vi "IOLINK LED STATE.vi"(7 "IP":string="192.168.23.100", 8 "error in (no error)":errorcluster) -> (0 "error out":errorcluster, 2 "MASTER STATUS":T2, 3 "JSON DATA - Payload":string)   [LabVIEW 2024]
uses:
  <vilib>/JDP Science/JSONtext/Find Item.vi
  <vilib>/JDP Science/JSONtext/String Subset.vi
  <vilib>/JDP Science/JSONtext/Offset/Find Object Item Locations by Names.vi
  <vilib>/JDP Science/JSONtext/support/Quote and Escape JSON string.vi
  <vilib>/JDP Science/JSONtext/Next JSON Value.vi
  <vilib>/JDP Science/JSONtext/Parsing/Advance past whitespace.vi
  <vilib>/JDP Science/JSONtext/support/Commas Needed.vi
  <vilib>/JDP Science/JSONtext/Parsing/Advance past whitespace and comma.vi
  <vilib>/JDP Science/JSONtext/Parsing/Advance past next JSON Value (inlined COPY).vi
  <vilib>/JDP Science/JSONtext/Parsing/Advance past Item Name.vi
  <vilib>/JDP Science/JSONtext/support/quote and escape json string 2.vi
  <vilib>/JDP Science/JSONtext/Parsing/Advance past Line Ending.vi
  <vilib>/JDP Science/JSONtext/Parsing/Advance past String.vi
  <vilib>/JDP Science/JSONtext/Parsing/Advance past Number.vi
  <vilib>/JDP Science/JSONtext/Parsing/Parse Full Path or Item Name.vi
  <vilib>/JDP Science/JSONtext/Parsing/Advance past Array.vi
  <vilib>/JDP Science/JSONtext/Parsing/Advance past Object.vi
  <vilib>/JDP Science/JSONtext/support/Error Cluster From Code.vi
  <vilib>/JDP Science/JSONtext/Offset/Find Item Locations by Path.vi
  <vilib>/JDP Science/JSONtext/Parsing/Parsing Error.vi
  <vilib>/JDP Science/JSONtext/JSONtext.lvlib
  <vilib>/NI/Advanced HTTP Client/Session.lvclass
panel:
  out "ON-offD 4":bool
  out "ON-offD 3":bool
  out "ON-offD 2":bool
  out "ON-offD":bool
  out "Statusd":bool
  out "Powerd":bool
  in  "MASTER STATUS 2":T1
  # "Master led status"
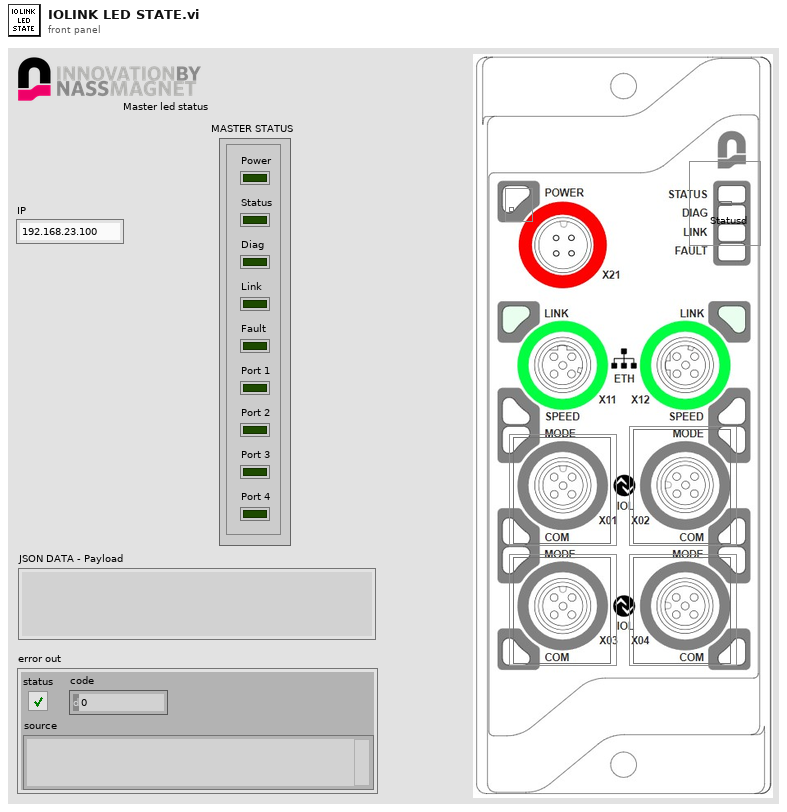
[diagram p1: front panel]
types:
  T1 = cluster{"Power":bool, "Status":bool, "Diag":bool, "Link":bool, "Fault":bool, "Port 1":bool, "Port 2":bool, "Port 3":bool, "Port 4":bool}
  T2 = cluster{"Power":bool, "Status":bool, "Diag":bool, "Link":bool, "Fault":bool, "Port 1":bool, "Port 3":bool, "Port 2":bool, "Port 4":bool}
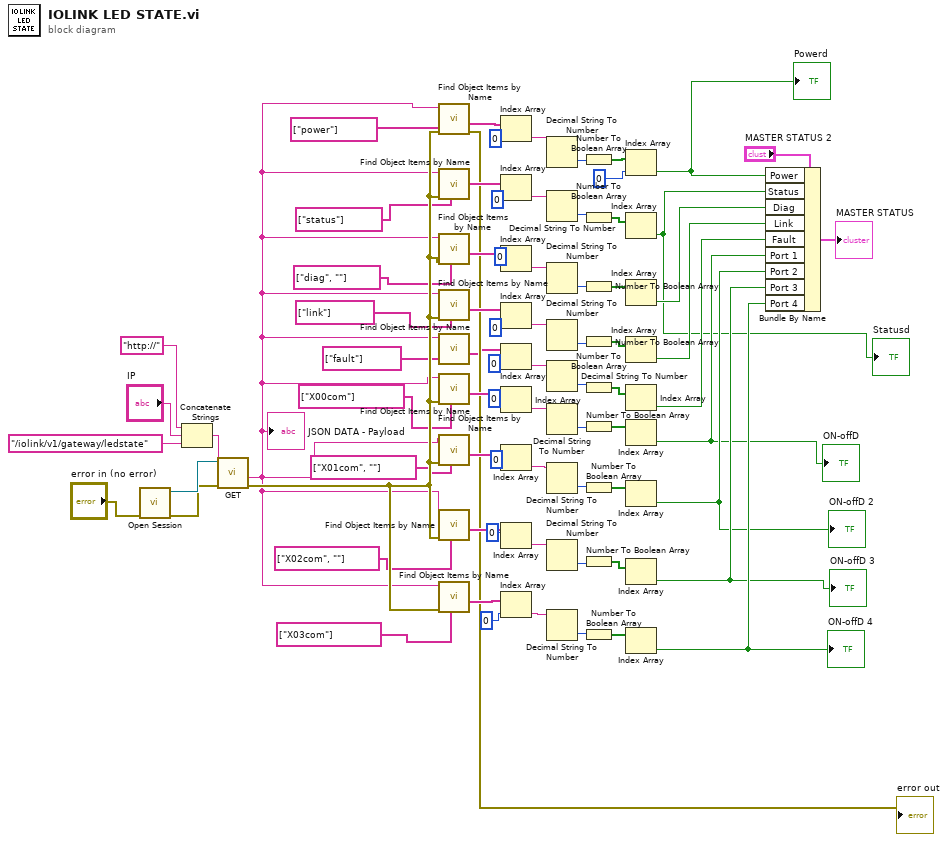
[diagram p0: block diagram]
diagram:
  n1 = call <vilib>:"Open Session.vi"("error in"="error in (no error)") -> ("error out"=w70:errorcluster, "session"=w72:refnum<class "Session.lvclass">)  [unwired: 9 in]
  n2 = Concatenate Strings("http://" ("url"), "IP", "/iolink/v1/gateway/ledstate" ("string")) -> (w71:string)
  n3 = call <vilib>:"GET.vi"("error in"=w70, "url"=w71, "session in"=w72) -> ("error out"=w66:errorcluster, "body"=w29:string)  [unwired: 4 in, 3 out]
  "JSON DATA - Payload" <- w29
  n4 = call <vilib>:"Find Object Items by Name.vi"("Item Names"=string[] ["power"], "error in (no error)"=w66, "JSON"=w29) -> ("error out"=→"error out":errorcluster, "<JSON>"=w69:string[])  [unwired: 6 in, 1 out]
  n5 = call <vilib>:"Find Object Items by Name.vi"("Item Names"=string[] ["status"] ("PWR 2"), "error in (no error)"=w66, "JSON"=w29) -> ("<JSON>"=w65:string[])  [unwired: 6 in, 2 out]
  n6 = call <vilib>:"Find Object Items by Name.vi"("Item Names"=string[] ["diag", ""] ("PWR 3"), "error in (no error)"=w66, "JSON"=w29) -> ("<JSON>"=w64:string[])  [unwired: 6 in, 2 out]
  n7 = call <vilib>:"Find Object Items by Name.vi"("Item Names"=string[] ["link"] ("PWR 4"), "error in (no error)"=w66, "JSON"=w29) -> ("<JSON>"=w63:string[])  [unwired: 6 in, 2 out]
  n8 = call <vilib>:"Find Object Items by Name.vi"("Item Names"=string[] ["fault"], "JSON"=w29) -> ("<JSON>"=w31:string[])  [unwired: 7 in, 2 out]
  n9 = call <vilib>:"Find Object Items by Name.vi"("Item Names"=string[] ["X00com"] ("PWR 5"), "error in (no error)"=w66, "JSON"=w29) -> ("<JSON>"=w62:string[])  [unwired: 6 in, 2 out]
  n10 = call <vilib>:"Find Object Items by Name.vi"("Item Names"=string[] ["X01com", ""] ("PWR 6"), "error in (no error)"=w66, "JSON"=w29) -> ("<JSON>"=w61:string[])  [unwired: 6 in, 2 out]
  n11 = call <vilib>:"Find Object Items by Name.vi"("Item Names"=string[] ["X02com", ""] ("PWR 7"), "error in (no error)"=w66, "JSON"=w29) -> ("<JSON>"=w60:string[])  [unwired: 6 in, 2 out]
  n12 = call <vilib>:"Find Object Items by Name.vi"("Item Names"=string[] ["X03com"] ("PWR 8"), "error in (no error)"=w66, "JSON"=w29) -> ("<JSON>"=w59:string[])  [unwired: 6 in, 2 out]
  n13 = Index Array(array=w69, index=0) -> (element=w67:string)
  n14 = Index Array(array=w65, index=0) -> (element=w58:string)
  n15 = Index Array(array=w64, index=0) -> (element=w57:string)
  n16 = Index Array(array=w63, index=0) -> (element=w56:string)
  n17 = Index Array(array=w31, index=0) -> (element=w30:string)
  n18 = Index Array(array=w62, index=0) -> (element=w55:string)
  n19 = Index Array(array=w61, index=0) -> (element=w54:string)
  n20 = Index Array(array=w60, index=0) -> (element=w53:string)
  n21 = Index Array(array=w59, index=0) -> (element=w52:string)
  n22 = Decimal String To Number(string=w67) -> (number=w28:i32)  [unwired: 2 in, 1 out]
  n23 = Decimal String To Number(string=w58) -> (number=w25:i32)  [unwired: 2 in, 1 out]
  n24 = Decimal String To Number(string=w57) -> (number=w24:i32)  [unwired: 2 in, 1 out]
  n25 = Decimal String To Number(string=w56) -> (number=w23:i32)  [unwired: 2 in, 1 out]
  n26 = Decimal String To Number(string=w30) -> (number=w22:i32)  [unwired: 2 in, 1 out]
  n27 = Decimal String To Number(string=w55) -> (number=w21:i32)  [unwired: 2 in, 1 out]
  n28 = Decimal String To Number(string=w54) -> (number=w20:i32)  [unwired: 2 in, 1 out]
  n29 = Decimal String To Number(string=w53) -> (number=w19:i32)  [unwired: 2 in, 1 out]
  n30 = Decimal String To Number(string=w52) -> (number=w18:i32)  [unwired: 2 in, 1 out]
  n31 = Number To Boolean Array(number=w28) -> (Boolean array=w27:bool[])
  n32 = Number To Boolean Array(number=w25) -> (Boolean array=w17:bool[])
  n33 = Number To Boolean Array(number=w24) -> (Boolean array=w16:bool[])
  n34 = Number To Boolean Array(number=w23) -> (Boolean array=w10:bool[])
  n35 = Number To Boolean Array(number=w22) -> (Boolean array=w11:bool[])
  n36 = Number To Boolean Array(number=w21) -> (Boolean array=w12:bool[])
  n37 = Number To Boolean Array(number=w20) -> (Boolean array=w13:bool[])
  n38 = Number To Boolean Array(number=w19) -> (Boolean array=w14:bool[])
  n39 = Number To Boolean Array(number=w18) -> (Boolean array=w15:bool[])
  n40 = Index Array(array=w27, index=0) -> (element=w2:bool)
  "Powerd" <- w2
  n41 = Index Array(array=w17) -> (element=w1:bool)  [unwired: 1 in]
  "Statusd" <- w1
  n42 = Index Array(array=w16) -> (element=w9:bool)  [unwired: 1 in]
  n43 = Index Array(array=w10) -> (element=w8:bool)  [unwired: 1 in]
  n44 = Index Array(array=w11) -> (element=w7:bool)  [unwired: 1 in]
  n45 = Index Array(array=w12) -> (element=w3:bool)  [unwired: 1 in]
  "ON-offD" <- w3
  n46 = Index Array(array=w13) -> (element=w4:bool)  [unwired: 1 in]
  "ON-offD 2" <- w4
  n47 = Index Array(array=w14) -> (element=w5:bool)  [unwired: 1 in]
  "ON-offD 3" <- w5
  n48 = Index Array(array=w15) -> (element=w6:bool)  [unwired: 1 in]
  "ON-offD 4" <- w6
  n49 = Bundle By Name(cluster="MASTER STATUS 2", "Power"=w2, "Status"=w1, "Diag"=w9, "Link"=w8, "Fault"=w7, "Port 1"=w3, "Port 2"=w4, "Port 3"=w5, "Port 4"=w6) -> (→"MASTER STATUS":T1)
